vi "PH_Cont-601k_PSU.connect to Device.vi"(0 "VI in":refnum<vi>, 5 "error in (no error)":errorcluster) -> (14 "VI out":refnum<vi>, 18 "Device Error out":errorcluster, 19 "error out":errorcluster)   [LabVIEW 2014, in "PH_Cont-601k_PSU.lvlib"]
uses:
  PH_Cont-601k_PSU.lvlib
  PH_Cont-601k_PSU.Device Informaton.ctl
  instr.lib/pu601k/Continuum PU610K.lvlib
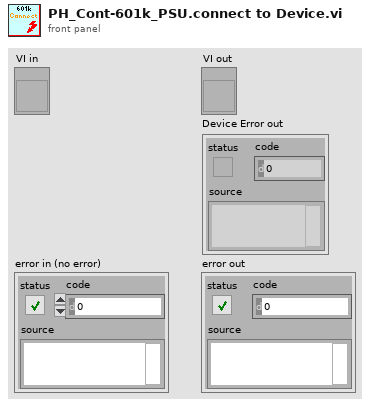
[diagram p1: front panel]
types:
  T1 = typedef "PH_Cont-601k_PSU.lvlib/PH_Cont-601k_PSU.Device Informaton.ctl" = cluster{"VISA resource":refnum<visa-resource-name>, "Driver Revision":string, "Firmware Revision":string}
  T2 = enum16{"Ch intl, Fl intl, QSw intl", "Ch intl, Fl intl, QSw ext", "Ch intl, Fl ext, QSw intl", "Ch intl, Fl ext, QSw ext", "Ch ext, Fl int, QSw int", "Ch ext, Fl int, QSw ext", "Ch ext, Fl ext, QSw int", "Ch ext, Fl ext, QSw ext"}
  T3 = typedef "PH_Cont-601k_PSU.lvlib/PH_Cont-601k_PSU.i attribute.ctl" = cluster{"GUI Refs":T4, "Interlock":bool, "Service ID applied Voltage":i32, "Device Settings":cluster{"Configuration":T5, "Flash Interval [s]":dbl, "Mode":T6, "Voltage [V]":u16, "Charge":bool, "VISA resource name":refnum<visa-resource-name>}, "Readyness":T7, "Information":cluster{"VISA resource name":refnum<visa-resource-name>, "Tagname Power On":string, "Interlock":cluster{"Instance":string, "Tagname":string}, "Limits [V]":cluster{"Lower":dbl, "Upper":dbl}, "Tagname PSU On":string}, "R2S":bool, "Charge is allowed":bool}
  T4 = typedef "PH_Cont-601k_PSU.lvlib/PH_Cont-601k_PSU.GUI Refs.ctl" = cluster{"Power On":refnum<vi>, "Hard- and Software":refnum<vi>, "Device Status":refnum<vi>, "Device Error":refnum<vi>, "Configuration":refnum<vi>, "Flash Interval [s]":refnum<vi>, "Interlock":refnum<vi>, "Interlock Indicator":refnum<vi>, "Voltage [V]":refnum<vi>, "Readyness":refnum<vi>, "Mode":refnum<vi>, "Reset Error":refnum<vi>, "Expert working":refnum<vi>, "Charge":refnum<vi>, "PSU On":refnum<vi>}
  T5 = typedef "PH_Cont-601k_PSU.lvlib/PH_Cont-601k_PSU.Configuration.ctl" = u16
  T6 = typedef "PH_Cont-601k_PSU.lvlib/PH_Cont-601k_PSU.Mode.ctl" = enum32{"STOP", "STANDBY", "READY", "EMISSION", "ERROR"}
  T7 = typedef "PH_Cont-601k_PSU.lvlib/PH_Cont-601k_PSU.Readyness.ctl" = cluster{"Program":T8, "Device":T9}
  T8 = typedef "PH_Cont-601k_PSU.lvlib/PH_Cont-601k_PSU.Readyness Program.ctl" = enum32{"OFF", "POWER", "INTERLOCK"}
  T9 = typedef "PH_Cont-601k_PSU.lvlib/PH_Cont-601k_PSU.Readyness Device.ctl" = enum32{"OFF", "CONNECTING", "CONNECTED", "OPERATING", "EOC", "ERROR"}
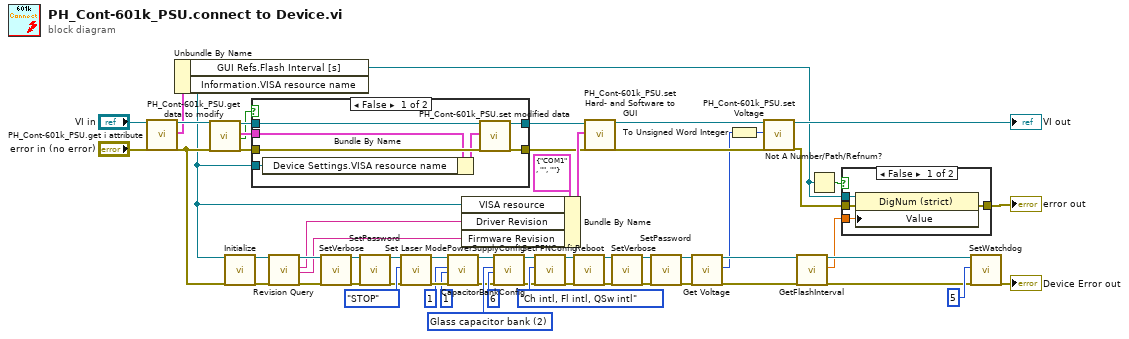
[diagram p0: block diagram]
diagram:
  w58 = u16 2 items=["Simmer capacitor bank"=1, "Glass capacitor bank"=2] ("type")
  n1 = call "PH_Cont-601k_PSU.get i attribute.vi"("i ref in"="VI in", "error in (no error)"="error in (no error)") -> ("i ref out"=w14:refnum<vi>, "i attribute"=w6:T3, "error out"=w32:errorcluster)  [unwired: 15 in]
  n2 = Unbundle By Name(w6) -> ("GUI Refs.Flash Interval [s]"=w4:refnum<vi>, "Information.VISA resource name"=w5:refnum<visa-resource-name>)
  n3 = call "PH_Cont-601k_PSU.get data to modify.vi"("i ref in"=w14, "error in (no error)"=w32) -> ("i ref out"=w13:refnum<vi>, "i attribute"=w12:T3, "timed out"=w10:bool, "error out"=w16:errorcluster)  [unwired: 14 in]
  n4 = call "Initialize.vi"("VISA resource name"=w5, "error in (no error)"=w32) -> ("VISA resource name out"=w35:refnum<visa-resource-name>, "error out"=w34:errorcluster)  [unwired: 16 in]
  n5 = case shown="False" w10 {
    tunnel: w16 -> [w67 w68]
    tunnel: [w66 w68] -> w15
    tunnel: w13 -> [w65 w69]
    tunnel: w12 -> [w64 _]
    tunnel: [w63 w69] -> w11
    tunnel: w5 -> [w61 _]
    frame False {
      n6 = Bundle By Name(cluster=w64, "Device Settings.VISA resource name"=w61) -> (w62:T3)
      n7 = call "PH_Cont-601k_PSU.set modified data.vi"("i ref in"=w65, "i attribute"=w62, "error in (no error)"=w67) -> ("i ref out"=w63:refnum<vi>, "error out"=w66:errorcluster)  [unwired: 15 in]
    }
    frame True {
    }
  }
  n8 = call "Revision Query.vi"("VISA resource name"=w35, "error in (no error)"=w34) -> ("VISA resource name out"=w37:refnum<visa-resource-name>, "Instrument Driver Revision"=w31:string, "Instrument Firmware Revision"=w30:string, "error out"=w39:errorcluster)  [unwired: 14 in]
  n9 = call "SetVerbose.vi"("VISA resource name"=w37, "error in"=w39) -> ("VISA resource name out"=w38:refnum<visa-resource-name>, "error out"=w40:errorcluster)  [unwired: 16 in]
  n10 = call "SetPassword.vi"("VISA resource name"=w38, "error in"=w40) -> ("VISA resource name out"=w50:refnum<visa-resource-name>, "error out"=w51:errorcluster)  [unwired: 16 in]
  n11 = call "Set Laser Mode.vi"("VISA resource name"=w50, "Mode"=enum16{"STOP", "STANDBY", "READY", "EMISSION"}."STOP", "error in"=w51) -> ("VISA resource name out"=w53:refnum<visa-resource-name>, "error out"=w52:errorcluster)  [unwired: 15 in]
  n12 = call "PowerSupplyConfig.vi"("VISA resource name"=w53, "Option Number"=1, "State"=1, "error in"=w52) -> ("VISA resource name out"=w55:refnum<visa-resource-name>, "error out"=w57:errorcluster)  [unwired: 14 in]
  n13 = Bundle By Name(cluster=T1 {"VISA resource"="COM1", "Driver Revision"="", "Firmware Revision"=""} ("Hard- and Software"), "VISA resource"=w5, "Driver Revision"=w31, "Firmware Revision"=w30) -> (w20:T1)
  n14 = call "CapacitorBankConfig.vi"("VISA resource name"=w55, "type"=w58, "number of capacitor banks"=6, "error in"=w57) -> ("VISA resource name out"=w56:refnum<visa-resource-name>, "error out"=w29:errorcluster)  [unwired: 14 in]
  n15 = call "SetPFNConfig.vi"("VISA resource name"=w56, "PFN Mode"=T2."Ch intl, Fl intl, QSw intl", "error in"=w29) -> ("VISA resource name out"=w43:refnum<visa-resource-name>, "error out"=w44:errorcluster)  [unwired: 15 in]
  n16 = call "Reboot.vi"("VISA resource name"=w43, "error in"=w44) -> ("VISA resource name out"=w45:refnum<visa-resource-name>, "error out"=w47:errorcluster)  [unwired: 16 in]
  n17 = call "PH_Cont-601k_PSU.set Hard- and Software to GUI.vi"("VI in"=w11, "Hard- and Software"=w20, "error in (no error)"=w15) -> ("VI out"=w19:refnum<vi>, "error out"=w28:errorcluster)  [unwired: 15 in]
  n18 = call "SetVerbose.vi"("VISA resource name"=w45, "error in"=w47) -> ("VISA resource name out"=w46:refnum<visa-resource-name>, "error out"=w48:errorcluster)  [unwired: 16 in]
  n19 = call "SetPassword.vi"("VISA resource name"=w46, "error in"=w48) -> ("VISA resource name out"=w25:refnum<visa-resource-name>, "error out"=w22:errorcluster)  [unwired: 16 in]
  n20 = call "Get Voltage.vi"("VISA resource name"=w25, "error in"=w22) -> ("VISA resource name out"=w26:refnum<visa-resource-name>, "voltage [V]"=w2:i32, "error out"=w23:errorcluster)  [unwired: 15 in]
  n21 = To Unsigned Word Integer(number=w2) -> (unsigned 16bit integer=w1:u16)
  n22 = call "PH_Cont-601k_PSU.set Voltage.vi"("VI in"=w19, "Voltage [V]"=w1, "error in (no error)"=w28) -> ("VI out"=→"VI out":refnum<vi>, "error out"=w3:errorcluster)  [unwired: 14 in, 1 out]
  n23 = call "GetFlashInterval.vi"("VISA resource name"=w26, "error in"=w23) -> ("VISA resource name out"=w24:refnum<visa-resource-name>, "interval (s)"=w18:dbl, "error out"=w21:errorcluster)  [unwired: 15 in]
  n24 = Not A Number/Path/Refnum?(number/path/refnum=w4) -> (NaN/Path/Refnum?=w17:bool)
  n25 = case shown="False" w17 {
    tunnel: w3 -> [w73 w74]
    tunnel: [w72 w74] -> w8
    tunnel: w4 -> [w71 _]
    tunnel: w18 -> [w70 _]
    frame False {
      n26 = property class="DigNum (strict)"(reference=w71, error in=w73, "Value"=w70) -> (error out=w72:errorcluster)  [unwired: 1 out]
    }
    frame True {
    }
  }
  "error out" <- w8
  n27 = call "SetWatchdog.vi"("VISA resource name"=w24, "watchdog time (1s)"=u16 5 ("watchdog time (s)"), "error in"=w21) -> ("error out"=→"Device Error out":errorcluster)  [unwired: 15 in, 1 out]
